vi "Milliseconds to seconds.vi"() -> ()   [LabVIEW 2018]
panel:
  out "out":dbl
  in  "in":dbl
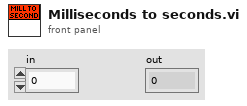
[diagram p1: front panel]
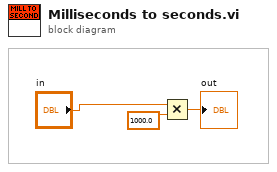
[diagram p0: block diagram]
diagram:
  n1 = Multiply(x="in", y=1000.0) -> (x*y=→"out":dbl)
